vi "AlliGator Fit Decay.vi"(0 "Selected Plot Info + Flag":T13={"Multiplot XY Graph"=refnum, "Mouse Coordinates"={"Horizontal"=0, "Vertical"=0}, "Plot Index"=-1, "Flag"=FALSE}, 1 "Decay Fit Options & Parameters":T2={"SYNC Period"=0.0, "Fit Options"={"Show Fit Residuals"=FALSE, "Fit Model"=enum."1-Exponential", "Residual Type"=enum."Standard", "Max Decay Percentile"=0.0, "Min Decay Percentile"=0.0, "Show Full Decay"=FALSE, "Weights"=enum."Unweighted", "Fitting Method"=enum."Least Square", "Compute Parameter Uncertainties"=FALSE, "Periodic Boundaries"=FALSE, "Model Calculation"=enum."Simulation", "Period"=0.0, "Termination Criteria"={"Max Iterations"=0, "Max Function Calls"=0, "Max Time"=0.0, "Function Tolerance"=0.0, "Parameter Tolerance"=0.0, "Gradient Tolerance"=0.0, "Min Lambda"=0.0, "Max Lambda"=0.0, "Initial Tick Count"=0}, "Offset Resolution"=0.0, "Use Local IRF"=FALSE, "Fitting Algorithm"=enum."Levenberg-Marquardt", "Show Confidence Interval "=TRUE, "Confidence Level"=95.0}, "Fit Parameter Constraints"=[], "MLE Baseline Offset"=0.0, "MLE Baseline Offset Type"=enum."Absolute"} {"Fit Options"."Confidence Level" min=0.0 max=100.0; "Fit Options"."Offset Resolution" min=0.0; "Fit Options"."Period" min=0.0; "Fit Options"."Min Decay Percentile" min=0.0 max=1.0; "Fit Options"."Max Decay Percentile" min=0.0 max=100.0; "Fit Parameter Constraints"."Max Value" format="%#.3g"; "Fit Parameter Constraints"."Min Value" format="%#.3g"}, 5 "Current Decay Name":string, 7 "Current Decay":T16, 9 "Reference Decay":T16, 11 "error in (no error)":errorcluster, 12 "Use Legacy Fitting Approach":bool) -> (2 "Decay Fit Options & Parameters (out)":T2={"SYNC Period"=0.0, "Fit Options"={"Show Fit Residuals"=FALSE, "Fit Model"=enum."1-Exponential", "Residual Type"=enum."Standard", "Max Decay Percentile"=0.0, "Min Decay Percentile"=0.0, "Show Full Decay"=FALSE, "Weights"=enum."Unweighted", "Fitting Method"=enum."Least Square", "Compute Parameter Uncertainties"=FALSE, "Periodic Boundaries"=FALSE, "Model Calculation"=enum."Simulation", "Period"=0.0, "Termination Criteria"={"Max Iterations"=0, "Max Function Calls"=0, "Max Time"=0.0, "Function Tolerance"=0.0, "Parameter Tolerance"=0.0, "Gradient Tolerance"=0.0, "Min Lambda"=0.0, "Max Lambda"=0.0, "Initial Tick Count"=0}, "Offset Resolution"=0.0, "Use Local IRF"=FALSE, "Fitting Algorithm"=enum."Levenberg-Marquardt", "Show Confidence Interval "=TRUE, "Confidence Level"=95.0}, "Fit Parameter Constraints"=[], "MLE Baseline Offset"=0.0, "MLE Baseline Offset Type"=enum."Absolute"} {"Fit Options"."Confidence Level" min=0.0 max=100.0; "Fit Options"."Offset Resolution" min=0.0; "Fit Options"."Period" min=0.0; "Fit Options"."Min Decay Percentile" min=0.0 max=1.0; "Fit Options"."Max Decay Percentile" min=0.0 max=100.0; "Fit Parameter Constraints"."Max Value" format="%#.3g"; "Fit Parameter Constraints"."Min Value" format="%#.3g"}, 3 "Fit Plots":T1, 4 "Best Fit Parameters (All)":dbl[](array[numeric]), 6 "Delta Best Fit Parameters (All)":dbl[](array[numeric]), 8 "R^2":dbl, 10 "Reduced Chi^2":dbl, 13 "Output Plot Names":string[](array[string]), 14 "Fit Output Message":string, 15 "Error Out":errorcluster)   [LabVIEW 2021, in "AlliGator Decay Fit.lvlib"]
doc: "VI implementing single decay fit with either a single or double exponential model with IRF convolution (or in the absence of IRF, without convolution)."
uses:
  AlliGator Decay Fit.lvlib
  <vilib>/Analysis/Matrix/Datatypes/RealMatrix.ctl
  Graphs/XY Graph/XY Graph Selected Plot Info+Flag.ctl
  Graphs/XY Graph/XY Graph Refnum.ctl
  <vilib>/Utility/miscctls.llb/LVPoint32TypeDef.ctl
  Decay Fit Parameter Map/AlliGator Decay Fit Options & Parameters v4.ctl
  Fits/IRF(X)PSED/Decay Fit Options v4.ctl
  Fits/Decay Convolution/Decay Model.ctl
  Fits/Residual Type.ctl
  Fits/IRF(X)PSED/Fit Weights Type v2.ctl
  Fits/Non-linear Fitting Method v2.ctl
  Fits/Fit Calculation Method.ctl
  Fits/Non-linear Fitting Algorithm.ctl
  AlliGator Decay Fit Parameter Constraints 2.ctl
  Fits/IRF(X)PSED/Decay Fit Parameters In List.ctl
  Fits/IRF(X)PSED/MLE Baseline Offset Type.ctl
  Fits/Fit Plots.ctl
  Settings/AlliGator Settings List.ctl
  Fits/Optimal Offset Selection Criterion.ctl
  Globals, Variables, Constants/AlliGator Variables List.ctl
  Fits/IRF(X)PSED/MLE Fit Options.ctl
  Graphs/LabVIEW Plot Interpolation.ctl
  Graphs/Get Plot at Mouse Click (XY Graph)/Get Plot at Mouse Click [AAC].vi
  <vilib>/Utility/error.llb/Error Cluster From Error Code.vi
  Fits/Decay Convolution/LM model function and gradient (1-Exp, Convolved, Periodic, Fixed Parameters) v3.vi
  Fits/Decay Convolution/LM model function and gradient (2-Exp, Convolved, Periodic, Fixed Parameters) v3.vi
  Fits/Abort Fit Global.vi
  <vilib>/ErrorRing/Error Ring.xnode
  Graphs/Graphs.lvlib
  Settings/AlliGator Settings.lvlib
  Graphs/XY Graph/XY Graph Add-Ons.lvlib
  Fits/Fits.lvlib
  Globals, Variables, Constants/AlliGator Globals, Variables & Constants.lvlib
  Time/Time.lvlib
  Strings/Strings.lvlib
  <vilib>/Analysis/Matrix/NI_Matrix.lvlib
  Decay Fit Parameter Map/AlliGator Decay Fit Parameter Map.lvlib
panel:
  in  "Reset Fit Options & Parameters":bool
  out "Covariance":T17
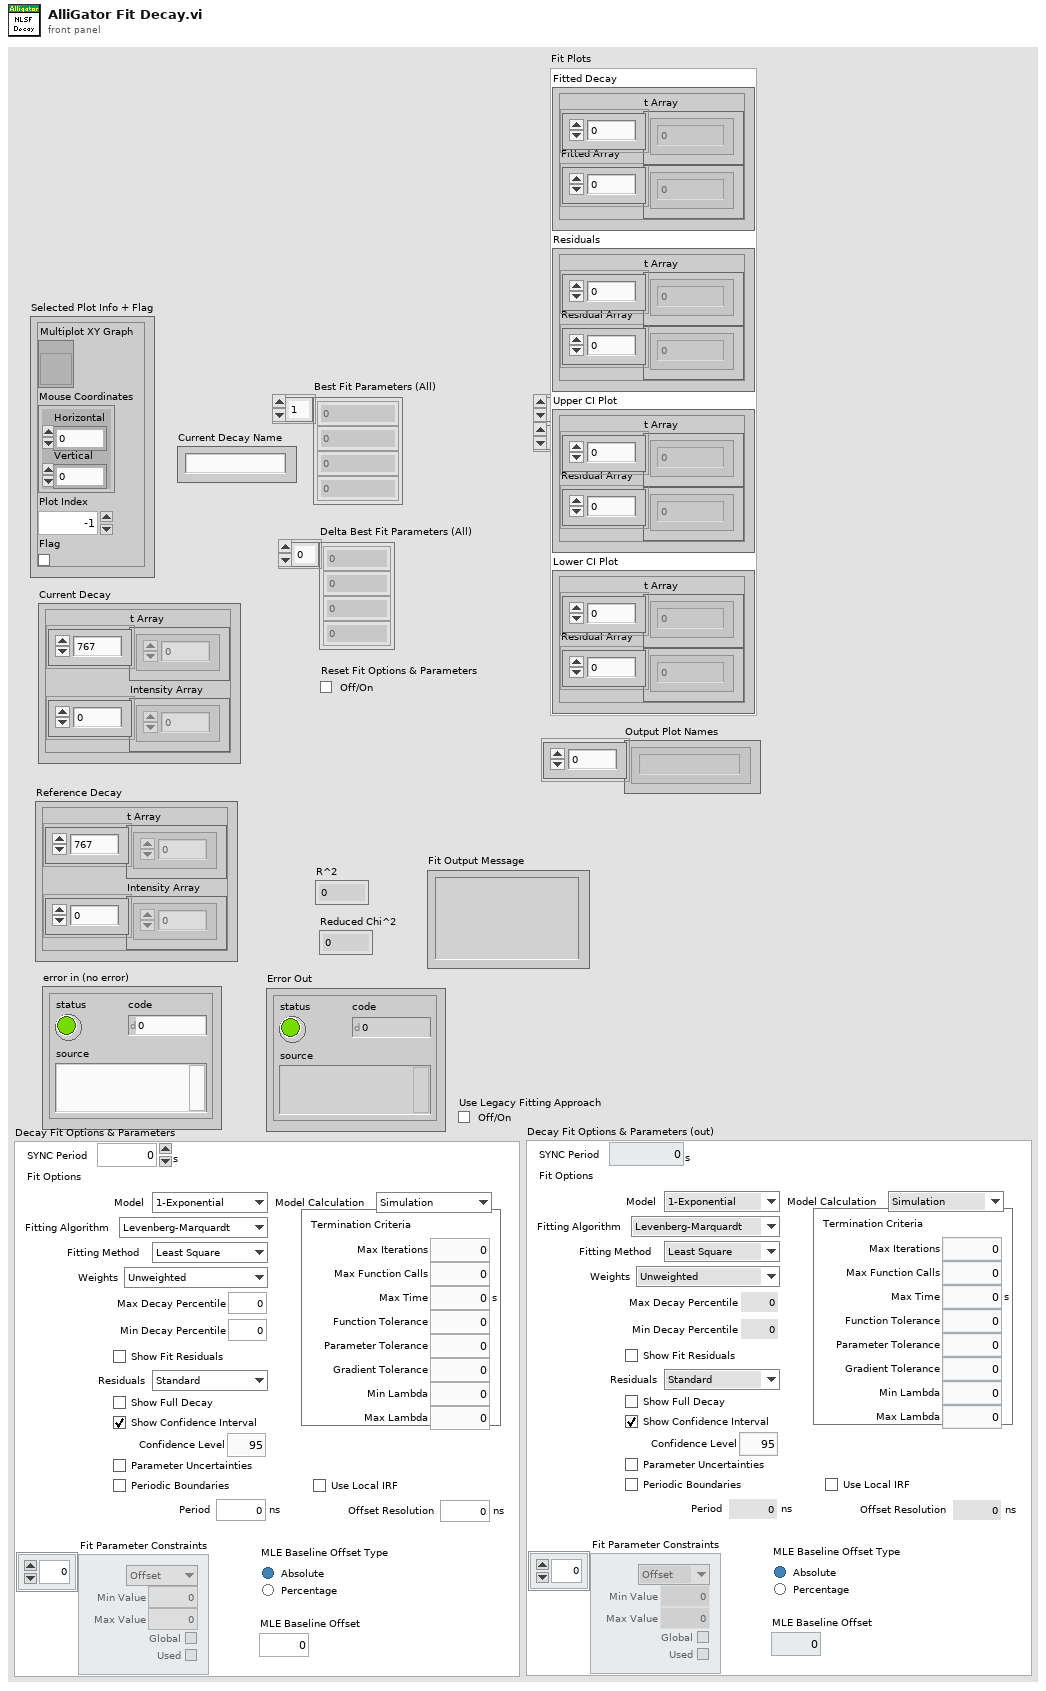
[diagram p1: front panel]
types:
  T1 = typedef "Fits.lvlib/Fit Plots.ctl" = cluster{"Fitted Decay":cluster{"t Array":dbl[], "Fitted Array":dbl[]}, "Residuals":cluster{"t Array":dbl[], "Residual Array":dbl[]}, "Upper CI Plot":cluster{"t Array":dbl[], "Residual Array":dbl[]}, "Lower CI Plot":cluster{"t Array":dbl[], "Residual Array":dbl[]}}
  T2 = typedef "AlliGator Decay Fit Parameter Map.lvlib/AlliGator Decay Fit Options & Parameters v4.ctl" = cluster{"SYNC Period":dbl[unit], "Fit Options":T3, "Fit Parameter Constraints":T10[], "MLE Baseline Offset":dbl, "MLE Baseline Offset Type":T12}
  T3 = typedef "Fits.lvlib/Decay Fit Options v4.ctl" = cluster{"Show Fit Residuals":bool, "Fit Model":T4, "Residual Type":T5, "Max Decay Percentile":dbl, "Min Decay Percentile":dbl, "Show Full Decay":bool, "Weights":T6, "Fitting Method":T7, "Compute Parameter Uncertainties":bool, "Periodic Boundaries":bool, "Model Calculation":T8, "Period":dbl[unit], "Termination Criteria":cluster{"Max Iterations":i32, "Max Function Calls":i32, "Max Time":dbl[unit], "Function Tolerance":dbl, "Parameter Tolerance":dbl, "Gradient Tolerance":dbl, "Min Lambda":dbl, "Max Lambda":dbl, "Initial Tick Count":u32}, "Offset Resolution":dbl[unit], "Use Local IRF":bool, "Fitting Algorithm":T9, "Show Confidence Interval ":bool, "Confidence Level":dbl}
  T4 = typedef "Fits.lvlib/Decay Model.ctl" = enum16{"1-Exponential", "2-Exponentials"}
  T5 = typedef "Fits.lvlib/Residual Type.ctl" = enum16{"Standard", "Normalized", "Reduced"}
  T6 = typedef "Fits.lvlib/Fit Weights Type v2.ctl" = enum16{"Unweighted", "1/Variance (Neyman)", "1/Variance (Pearson)", "Best of All"}
  T7 = typedef "Fits.lvlib/Non-linear Fitting Method v2.ctl" = enum16{"Least Square", "Least Absolute Residual", "Bisquare", "MLE", "-", "Best of All"}
  T8 = typedef "Fits.lvlib/Fit Calculation Method.ctl" = enum16{"Simulation", "Convolution", "Integration"}
  T9 = typedef "Fits.lvlib/Non-linear Fitting Algorithm.ctl" = enum16{"Levenberg-Marquardt", "Trust-Region Dogleg"}
  T10 = typedef "AlliGator Decay Fit.lvlib/AlliGator Decay Fit Parameter Constraints 2.ctl" = cluster{"Fit Parameter":T11, "Min Value":dbl, "Max Value":dbl, "Global":bool, "Used":bool}
  T11 = typedef "Fits.lvlib/Decay Fit Parameters In List.ctl" = enum16{"Offset", "Baseline", "A_1", "tau_1", "A_2", "tau_2"}
  T12 = typedef "Fits.lvlib/MLE Baseline Offset Type.ctl" = enum32{"Absolute", "Percentage"}
  T13 = typedef "XY Graph Add-Ons.lvlib/XY Graph Selected Plot Info+Flag.ctl" = cluster{"Multiplot XY Graph":T14, "Mouse Coordinates":T15, "Plot Index":i32, "Flag":bool}
  T14 = typedef "XY Graph Add-Ons.lvlib/XY Graph Refnum.ctl" = refnum<vi>
  T15 = typedef "LVPoint32TypeDef.ctl" = cluster{"Horizontal":i32, "Vertical":i32}
  T16 = cluster{"t Array":dbl[], "Intensity Array":dbl[]}
  T17 = typedef "NI_Matrix.lvlib/RealMatrix.ctl" = dbl[][]
  T18 = typedef "Fits.lvlib/Optimal Offset Selection Criterion.ctl" = enum16{"Min Chi^2", "Max R^2"}
  T19 = typedef "AlliGator Settings.lvlib/AlliGator Settings List.ctl" = enum16{"GUI:Visible Settings Tab", "GUI:Last Run Version", "Source Image:Use Image Histogram for Contrast", "Source Image:Low Count Pixels Rejection Options", "Source Image:High Count Pixels Rejection Options", "Source Image:Use Image Brightness", "Source Image:Blend Overlay with Image Background", "Source Image:Use Fixed ROI Diameter", "Source Image:ROI Diameter", "Source Image:ROI Center Color", "Source Image:Peak Threshold", "Source Image:Intensity Threshold", "Source Image:Image Binning Options", "Source Image:Image Smoothing Options", "Source Image:Image Histogram Active", "Source Image:Invert Binary Mask", "Source Image:Hot Pixel Removal", "Source Image:Overlay Analyzed ROI Center", "Source Image:Auto-Adjust Contrast", "Source Image:Histogram Lower Percentile", "Source Image:Histogram Upper Percentile", "Source Image:Save Source Image", "Source Image:Scale Bar Options", "Source Image:Image Resolution (Pixel Size)", "Source Image:Flatfield Correction", "Source Image:Show Dead Left Columns Correction", "Source Image:Dead Left Columns Correction", "Source Image:Image Pre-Processing Operations Order", "Source Image:Overlay ROI Median", "Source Image:Median Overlay Color", "Data Information:Gate Width", "Data Information:Nanotime Gate Separation", "Data Information:Macrotime Gate Separation", "Data Information:Gate Step", "Data Information:# Gates", "Data Information:Gate Image Exposure", "Data Information:Gate Image Integration", "Data Information:Gates to Skip", "Data Information:Gates to Keep", "Data Information:Define Gates to", "Data Information:Channel Name", "Data Information:Available Channel Names", "Data Information:Channel Arithmetic", "Data Information:Background File Subtraction", "Data Information:Background File", "Data Information:Background Scaling Factor", "Data Information:Background Pile-up Correction", "Data Information:Background Pixel Well Capacity", "Data Information:Laser Period", "Data Information:SYNC Period", "Data Information:Pile-up Correction", "Data Information:Pixel Well Capacity", "Data Information:Dataset Scaling Factor", "Fluorescence Decay_Decay Pre-Processing:Reverse Gates", "Fluorescence Decay_Decay Pre-Processing:Verbose Decay Pre-Processing", "Fluorescence Decay_Decay Pre-Processing:Use Decay Pre-Processing", "Fluorescence Decay_Decay Pre-Processing:Background Subtraction", "Fluorescence Decay_Decay Pre-Processing:Background Definition Range", "Fluorescence Decay_Decay Pre-Processing:Baseline Subtraction Method", "Fluorescence Decay_Decay Pre-Processing:Decay Pre-Processing Operations Order", "Fluorescence Decay_Decay Pre-Processing:Smoothing Parameter", "Fluorescence Decay_Decay Pre-Processing:Shift Decay", "Fluorescence Decay_Decay Pre-Processing:Decay Shift Parameters", "Fluorescence Decay_Decay Pre-Processing:Fold Decay", "Fluorescence Decay_Decay Pre-Processing:# Folds", "Fluorescence Decay_Decay Pre-Processing:1-Normalize Decay", "Fluorescence Decay_Decay Pre-Processing:[0-1]-Normalize Decay", "Fluorescence Decay_Decay Pre-Processing:Smoothen Decay", "Fluorescence Decay_Decay Pre-Processing:Extrapolate Decay", "Fluorescence Decay_Decay Pre-Processing:Use Periodicity", "Fluorescence Decay_Decay Pre-Processing:Use Cursors", "Fluorescence Decay_Decay Pre-Processing:Tail Fraction", "Fluorescence Decay_Decay Pre-Processing:Head Fraction", "Fluorescence Decay_Decay Pre-Processing:Additional Points", "Fluorescence Decay_Decay Pre-Processing:Straighten Decay", "Fluorescence Decay_Decay Pre-Processing:Constant Background", "Fluorescence Decay_Decay Pre-Processing:Pixel-Normalize Decay", "Fluorescence Decay_Advanced Analysis:Extract IRF instead of Decay", "Fluorescence Decay_Advanced Analysis:IRF Extraction Options", "Fluorescence Decay_Advanced Analysis:IRF Optimization Options", "Fluorescence Decay_Advanced Analysis:Square Pulse Options", "Fluorescence Decay_Advanced Analysis:IRF Order", "Fluorescence Decay_Advanced Analysis:IRF Time Constants", "Fluorescence Decay_Advanced Analysis:Wavelet Analysis Options", "Fluorescence Decay_Advanced Analysis:Average Lifetime Options", "Fluorescence Decay_Fit Options:Fit Options", "Fluorescence Decay_Fit Options:Use Legacy Fitting Approach", "Fluorescence Decay_Fit Options:Use Data Information Laser Period", "Fluorescence Decay_Fit Parameters:Displayed Fit Parameters", "Fluorescence Decay_Fit Parameters:Fit Parameter Constraints", "Fluorescence Decay_Fit Parameters:Export Tabulated Results", "Fluorescence Decay_Fit Parameters:MLE Baseline Offset Type", "Fluorescence Decay_Fit Parameters:MLE Baseline Offset", "Fluorescence Decay_Fit Parameters:Guess Parameter Names", "Fluorescence Decay_Fit Parameters:Guess Parameter Values", "Fluorescence Decay_Fit Parameters:Guess Parameters Options", "Fluorescence Decay_Fit Parameters:Optimal Offset Selection Criterion", "Fluorescence Decay_Styles:Show Last Decay Only", "Fluorescence Decay_Styles:Decay Graph Color Array", "Fluorescence Decay:Decay Graph Active", "Fluorescence Decay Statistics:Min Peak Value", "Fluorescence Decay Statistics:Reject Low Decay Peak Pixels", "Fluorescence Decay Statistics:Reject High Decay Peak Pixels", "Fluorescence Decay Statistics:Max Peak Value", "Time Traces:Use File Timestamp", "Time Traces:Time Step", "Time Traces:Use Intensity Correction File", "Time Traces:Intensity Correction File", "Phasor Plot:Phasor Plot Smoothing Options", "Phasor Plot:Phasor Plot Size", "Phasor Plot:Phasor Plot Graphics Options", "Phasor Plot:Cumulative Phasor Plot", "Phasor Plot:Use Phasor Brightness", "Phasor Plot:Blend Overlay with Phasor Background", "Phasor Plot:Save Phasor Plot", "Phasor Plot:Show References", "Phasor Plot:Phasor Ratio Decay Range", "Phasor Plot:Exponential Fading", "Phasor Plot:Phasor Ratio Reference Colors", "Phasor Plot:Reference Radius", "Phasor Plot:Show Color Map Vertices", "Phasor Plot:Phasor Plot Active", "Phasor Plot:Phasor Ratio Color Map Type", "Phasor Plot:Phasor Ratio Color Map", "Phasor Plot:Phasor Ratio Display Range", "Phasor Plot:Selected Image ROI(s)", "Phasor Plot:All Image ROIs", "Phasor Plot:Selected Phasor Plot ROI(s)", "Phasor Plot:All Phasor Plot ROIs", "Phasor Plot:Phasor Ratio Color-Coded Quantity", "Phasor Plot:Store Phasor Harmonics", "Phasor Plot:Draw Reference Segment", "Phasor Plot:User-Defined Quantity", "Phasor Plot:Color Scale High Color", "Phasor Plot:Color Scale Low Color", "Phasor Plot:Intensity-weighted Phasor Plot", "Phasor Graph:Phasor Frequency", "Phasor Graph:Phasor Ratio Type", "Phasor Graph:Pixel-level Phasor Computation", "Phasor Graph:Save Phasor Graph", "Phasor Graph:Phasor Graph Active", "Phasor Graph:Phasor SDV Options", "Phasor Graph:Intensity-weighted Phasor Graph", "Phasor Graph:Define Shortest Lifetime as", "Phasor Calibration:Use Backup Calibration if needed", "Phasor Calibration:Backup Calibration Type", "Phasor Calibration:Calibration Type", "Phasor Calibration:Calibration Lifetime", "Phasor Calibration:Calibration Map Algorithm", "Single-Exponential Phasor Locus (SEPL):Gate Parameters", "Single-Exponential Phasor Locus (SEPL):User-defined Gate", "Single-Exponential Phasor Locus (SEPL):User-defined IRF", "Single-Exponential Phasor Locus (SEPL):Phasor Parameters", "Single-Exponential Phasor Locus (SEPL):Decay & IRF Parameters", "Single-Exponential Phasor Locus (SEPL):Display Parameters", "Lifetime Analysis:Decay Analysis Parameters", "Lifetime Analysis:Lifetime Map Active", "Plugins:Python Settings", "Miscellaneous:Verbose Mode", "Miscellaneous:Beep after Script", "Miscellaneous:Saved Image File Format", "Miscellaneous:Exported Gate Image Settings", "Miscellaneous:Include Loading in Timing", "Miscellaneous:Verbose Settings Mode", "Miscellaneous:Histogram Options", "Miscellaneous:Beep on Error", "Miscellaneous:# Logical Processors Used", "Miscellaneous:ROI Description Max Characters", "Miscellaneous:Verbose Error Mode", "Miscellaneous:Transparent Mask Color"}
  T20 = typedef "XY Graph Add-Ons.lvlib/XY Graph Plot Data.ctl" = cluster{"X Array":dbl[], "Y Array":dbl[]}
  T21 = typedef "AlliGator Globals, Variables & Constants.lvlib/AlliGator Variables List.ctl" = enum16{"---- GUI ----", "GUI:Initialization Status", "GUI:State Indicators Refnum", "GUI:Original AlliGator Menu Items", "GUI:Current Action Loop State", "GUI:Script in progress", "GUI:Playback", "GUI:Loop Playback", "GUI:Search ROI Used", "GUI:Search ROI", "Decay Graph Max Legend Size", "Intensity Graph Max Legend Size", "Decay Statistics Graph Max Legend Size", "Phasor Graph Max Legend Size", "Phasor Ratio Graph Max Legend Size", "Lifetime Graph Max Legend Size", "---- Files ----", "Files:Export Dataset Frames as Individual Files", "Files:Show Batch Export Help Balloons", "Files:Frames in Dataset", "Files:ptu File Frame Start Indices", "Files:Current Frame in Dataset", "Files:Current Frame Timestamp", "Files:Dataset Loaded", "Files:Dataset Metadata", "Files:Dataset Channel", "Files:Dataset Data Description", "Files:Background Dataset Metadata", "Files:Background Dataset Channel", "Files:Background Dataset Data Description", "Files:Background File Subtraction", "Files:Background File Path", "Files:Background File Pile-up Correction", "Files:Background File Pixel Well Capacity", "Files:Background File Scaling Factor", "Files:Current Dataset Load Settings", "Files:Dataset Path", "Files:ICCD-specific Information", "Files:Macrotime Gate Separation", "------ Python Plugins ------", "Python Plugins:Information", "Python Plugins:Python Session", "Python Plugins:Valid Python Session?", "---- Source Image ----", "Source Image:ROIs", "Source Image:Current ROI", "Source Image:ROI Event Refnum", "X_Source Image:Display Range", "X_Source Image:Palette Information", "X_Source Image:Type of Displayed Image", "X_Time Gate Slider", "Source Image:Palette List", "Source Image:Scale", "Source Image:ROI Overlay Color", "Source Image:Overlay to Erase", "Source Image:Is Displayed Image Accumulated", "Source Image:White Light Image Modified", "Source Image:Mask Image Modified", "---- Image Profile Window ----", "Image Profile:Window Event Refnum", "Image Profile:IntensityType", "Image Profile:Intensity Average Type", "Image Profile:Intensity-weighted SDV", "Image Profile:Box Profile Type", "Image Profile:Window Open", "Image Profile:Plotted Fit Parameter", "------ Phasor Graph -------", "Phasor Graph:Show Line", "---- Phasor Plot ---", "Phasor Plot:Parameters Changed", "Phasor Plot:FLI Dataset Modified since last Calculation", "Phasor Harmonics Data", "Selected Phasor Harmonics", "Phasor Harmonic Manager Event Refnum", "Phasor Plot:ROIs", "Phasor Plot:Current ROI", "Phasor Plot:ROI Event Refnum", "Phasor Plot:Image Reference Points", "Phasor Plot:Computed", "Phasor Plot:Palette Information", "Phasor Plot:Palette List", "Phasor Plot:Phasor Ratio Palette Information", "Phasor Plot:Phasor Ratio Palette List", "Phasor Plot:Image Scale", "Phasor Plot:Image Overlay to Erase", "Phasor Plot:Image Elements to Update", "Phasor Plot:Current Calculation Parameters", "Phasor Plot:Current Calibration Options", "Phasor Plot:Reset Cumulated Phasor Plot", "Phasor Plot:Reference 1", "Phasor Plot:Lifetime Reference 1", "Phasor Plot:Reference 1 Frequency", "Phasor Plot:Reference 2", "Phasor Plot:Lifetime Reference 2", "Phasor Plot:Reference 2 Frequency", "---- Decay Analysis ----", "Number of Selected Decays to Fit", "LS Fit Results", "LAR Fit Results", "BS Fit Results", "Last Decay Max - Min", "Best Fit Parameters", "Best Fit Parameter Names", "Actual Size X", "Actual Size Y", "Binning X", "Binning Y", "Actual # Gates", "Dataset Number", "Gates to...", "Gates Skipped", "Gates to keep", "Gate Step", "Gate Separation", "Reversed Gates", "Pile-up Correction", "Pixel Well Capacity", "Background Subtracted", "Background Subtraction Method", "Background Definition Range", "Background File (deprecated)", "Number of Dataset Accumulated", "Array of Accumulated Dataset Paths", "Do Averaged Datasets", "Destination File Path", "Process Plot Target", "Use 1/D as Phasor Frequency", "---- Decay Fit Parameter Map -----", "Decay Fit Parameter Map:Palette Information", "Decay Fit Parameter Map:Palette List", "Decay Fit Parameter Map:X Resolution", "Decay Fit Parameter Map:Y Resolution", "Decay Fit Parameter Map:Use Decay Fit Result Constraints", "Decay Fit Parameter Map:Decay Fit Result Constraints", "Decay Fit Parameter Map:Decay Fit Result Constraints Applied", "---- Parameter Map ----", "Parameter Map:Palette Information", "Parameter Map:Palette List", "------- Local Decay Window ---------", "Local Decay Graph Window:Event Refnum", "Local Decay Graph Window:Use normalized IRF for convolution", "----- Miscellaneous ----", "Misc:Skippable Dialog Windows Status"}
  T22 = typedef "Fits.lvlib/MLE Fit Options.ctl" = cluster{"MLE Baseline Offset":dbl, "MLE Baseline Offset Type":T12}
  T23 = typedef "Fits.lvlib/Decay Fit Parameter Constraints Arrays.ctl" = cluster{"Parameter Bounds (Fix+Fit)":cluster{"parameter minimum":dbl[], "parameter maximum":dbl[]}, "Fitted Parameters":T11[], "Fixed Parameters":T11[], "Fit Model":T4}
  T24 = typedef "Graphs.lvlib/Plot Range.ctl" = cluster{"X Minimum":dbl, "X Maximum":dbl, "Y Minimum":dbl, "Y Maximum":dbl}
  T25 = cluster{"parameter minimum":dbl[], "parameter maximum":dbl[]}
  T26 = typedef "Fits.lvlib/Non-linear Fit Output v4.ctl" = cluster{"best nonlinear fit":dbl[], "best fit parameters":dbl[], "R^2":dbl, "RMSE":dbl, "error out":errorcluster, "Fitting Method":T27, "number of function calls":i32, "number of iterations":i32, "covariance":T17, "Chi 2":dbl, "DOF":i32, "Fit Convergence Criterion":T28, "Fitting Algorithm":T9, "Weighted Fit":T6, "Gradient":dbl, "|Delta Chi 2|":dbl, "|Delta Chi 2|/Chi 2":dbl, "Max |Delta a| /|a|":dbl, "Lambda":dbl, "RSS":dbl, "AIC":dbl, "BIC":dbl, "Max number of function calls":i32, "Max number of iterations":i32, "IRF":T20, "IRF Normalization Factor":dbl, "Decay Normalization Factor":dbl, "Number of offset fits":i32, "Weighted Chi2":dbl, "Unweighted Chi2":dbl}
  T27 = typedef "Fits.lvlib/Nonlinear Fit Method.ctl" = enum16{"Least Square", "Least Absolute Residual", "Bisquare", "MLE"}
  T28 = typedef "Fits.lvlib/Convergence Criteria.ctl" = enum16{"Continue", "Tolerances Exceeded", "Max Time Exceeded", "Max Iterations Exceeded", "Max Function Evaluations Exceeded", "Scale Range Exceeded"}
  T29 = typedef "AlliGator Decay Fit.lvlib/AlliGator Guess Parameters Options.ctl" = enum16{"Numerically estimated", "User-provided", "User-provided (normalized)", "Last valid fitted parameters"}
  T30 = typedef "Fits.lvlib/Fit Control Data v2.ctl" = cluster{"IRF":T20, "Laser Period":dbl, "SYNC Period":dbl, "Fixed Parameter Names":T11[], "Fixed Parameter Values":dbl[], "Fitted Parameter Names":T11[], "Fit Model":T4}
  T31 = typedef "Graphs.lvlib/LabVIEW Plot Interpolation.ctl" = enum16{"Point (.)", "Stepwise Right (--.)", "Line + Point (\\. /)", "Stepwise Left (.--)", "Stepwise Centered (-.-)", "Stepwise Vertical (|.|)", "Line (-)", "Use Previous Plot's Style"}
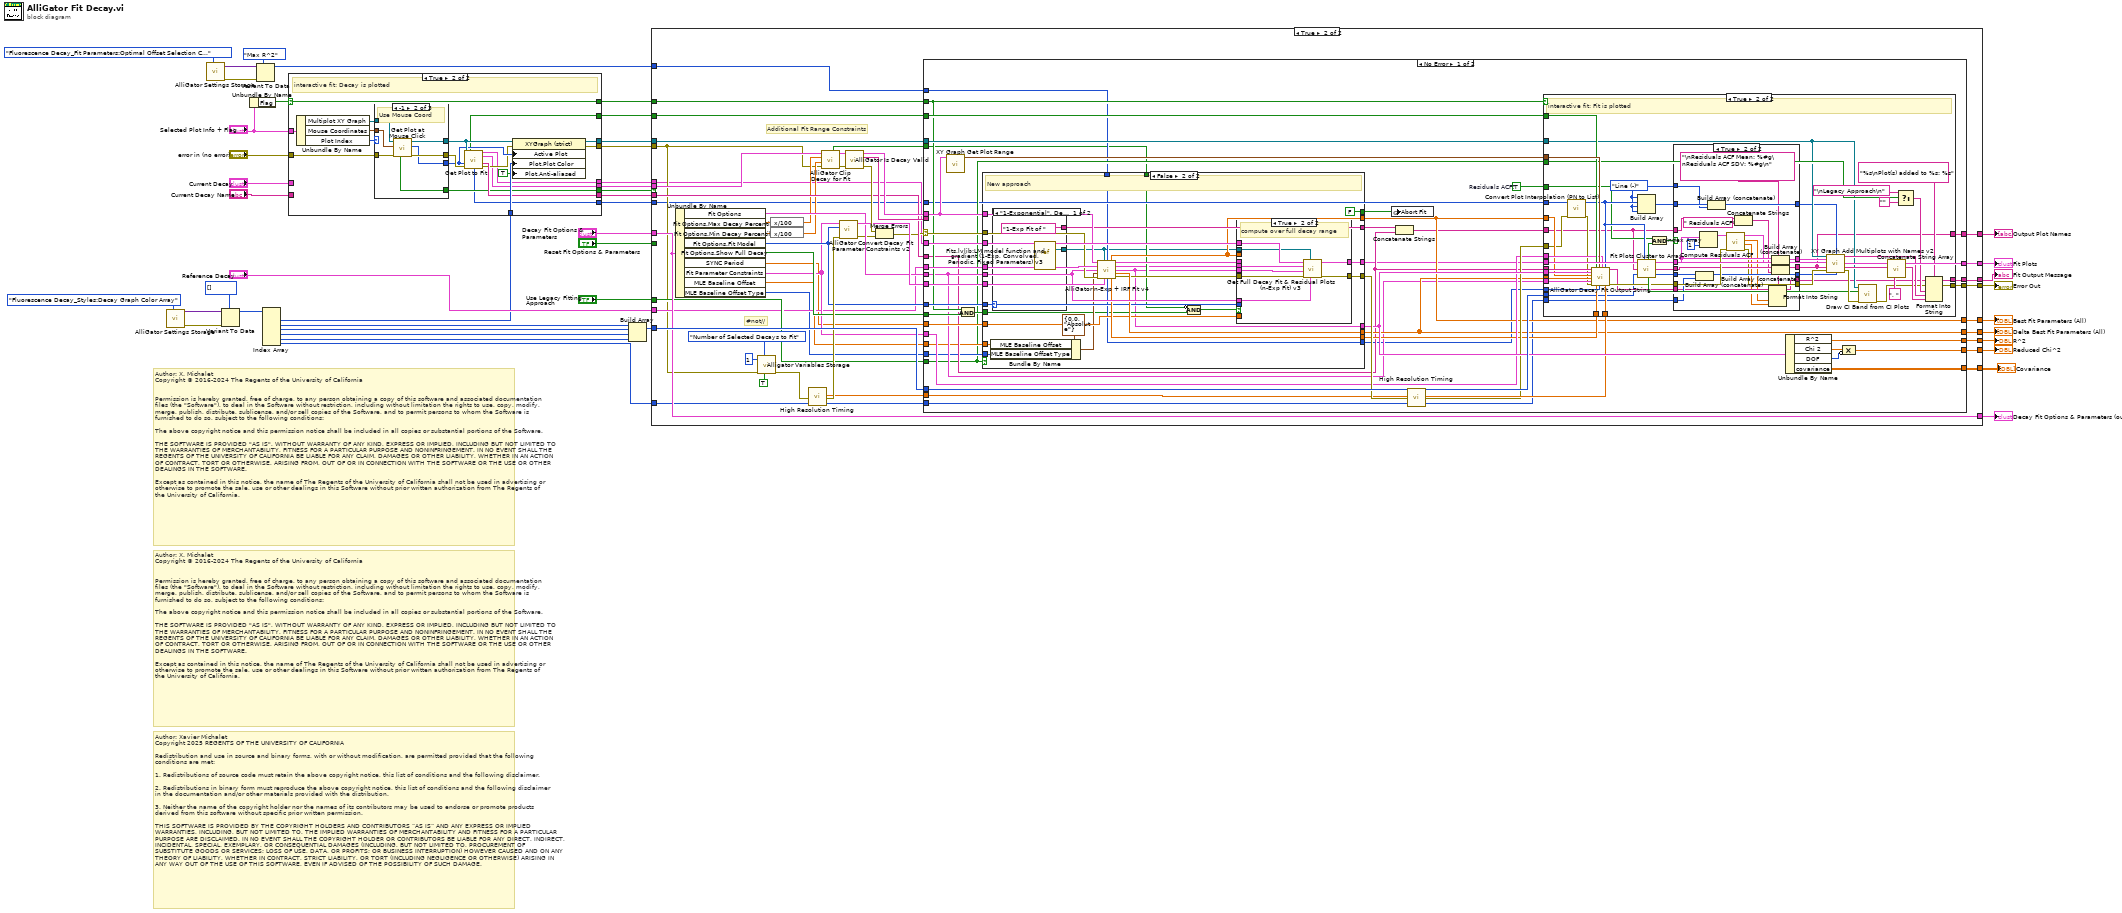
[diagram p0: block diagram]
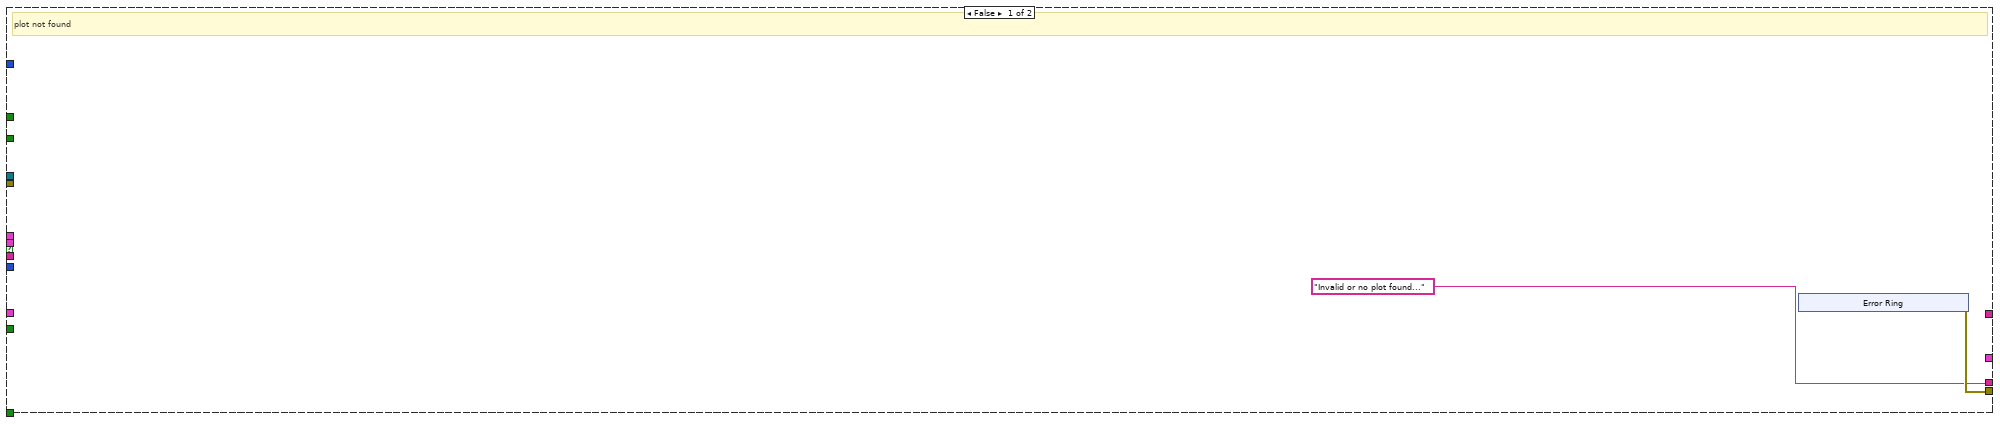
[diagram p2: hidden frame]
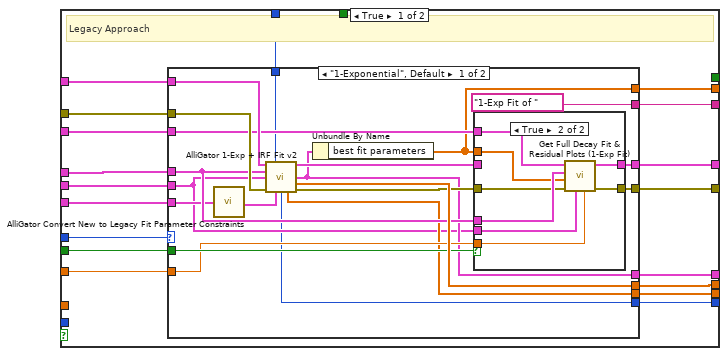
[diagram p5: hidden frame]
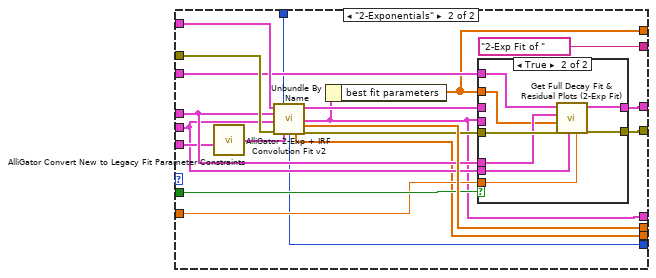
[diagram p7: hidden frame]
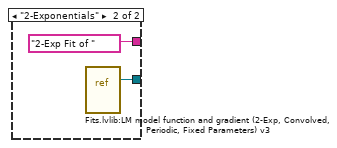
[diagram p9: hidden frame]
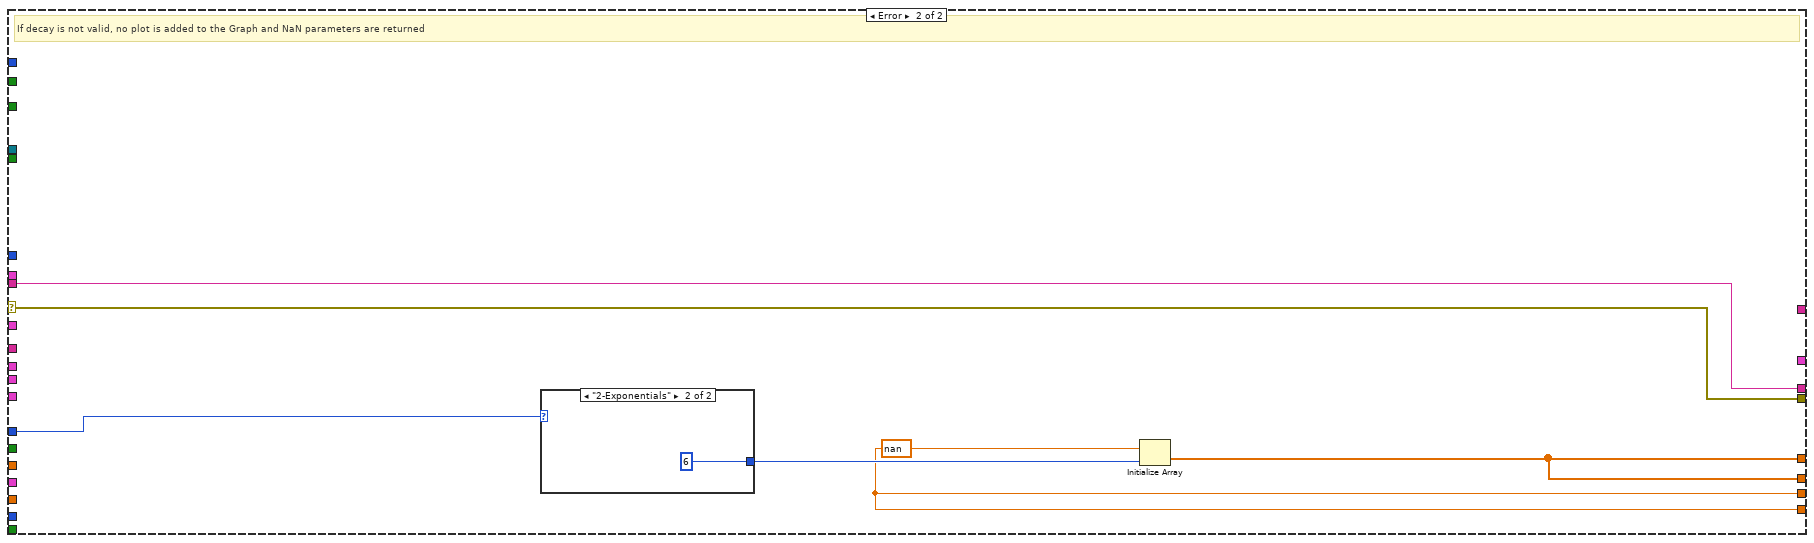
[diagram p11: hidden frame]
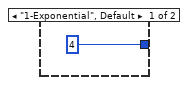
[diagram p12: hidden frame]
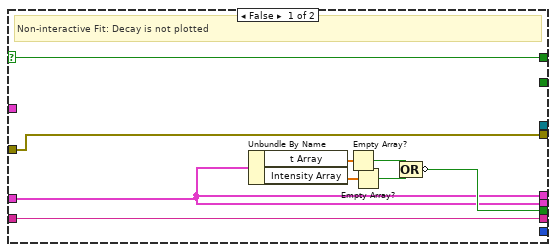
[diagram p13: hidden frame]
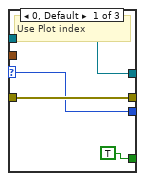
[diagram p14: hidden frame]
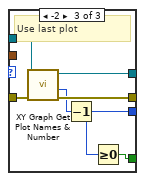
[diagram p15: hidden frame]
diagram:
  # "Author: Xavier Michalet\nCopyright 2025 REGENTS OF THE UNIVERSITY OF CALIFORNIA\n\nRedistribution and use in source and binary forms, with or without modification, are permitted provided that the following conditions are met:\n\n1. Redistributions of source code must retain the above copyright notice, this list of conditions and the following disclaimer.\n\n2. Redistributions in binary form must reproduce the above copyright notice, this list of conditions and the following disclaimer in the documentation and/or other materials provided with the distribution.\n\n3. Neither the name of the copyright holder nor the names of its contributors may be used to endorse or promote products derived from this software without specific prior written permission.\n\nTHIS SOFTWARE IS PROVIDED BY THE COPYRIGHT HOLDERS AND CONTRIBUTORS “AS IS” AND ANY EXPRESS OR IMPLIED WARRANTIES, INCLUDING, BUT NOT LIMITED TO, THE IMPLIED WARRANTIES OF MERCHANTABILITY AND FITNESS FOR A PARTICULAR PURPOSE ARE DISCLAIMED. IN NO EVENT SHALL THE COPYRIGHT HOLDER OR CONTRIBUTORS BE LIABLE FOR ANY DIRECT, INDIRECT, INCIDENTAL, SPECIAL, EXEMPLARY, OR CONSEQUENTIAL DAMAGES (INCLUDING, BUT NOT LIMITED TO, PROCUREMENT OF SUBSTITUTE GOODS OR SERVICES; LOSS OF USE, DATA, OR PROFITS; OR BUSINESS INTERRUPTION) HOWEVER CAUSED AND ON ANY THEORY OF LIABILITY, WHETHER IN CONTRACT, STRICT LIABILITY, OR TORT (INCLUDING NEGLIGENCE OR OTHERWISE) ARISING IN ANY WAY OUT OF THE USE OF THIS SOFTWARE, EVEN IF ADVISED OF THE POSSIBILITY OF SUCH DAMAGE."
  # "Author: X. Michalet\nCopyright © 2016-2024 The Regents of the University of California\n \n\nPermission is hereby granted, free of charge, to any person obtaining a copy of this software and associated documentation files (the \"Software\"), to deal in the Software without restriction, including without limitation the rights to use, copy, modify, merge, publish, distribute, sublicense, and/or sell copies of the Software, and to permit persons to whom the Software is furnished to do so, subject to the following conditions:\n\nThe above copyright notice and this permission notice shall be included in all copies or substantial portions of the Software.\n\nTHE SOFTWARE IS PROVIDED \"AS IS\", WITHOUT WARRANTY OF ANY KIND, EXPRESS OR IMPLIED, INCLUDING BUT NOT LIMITED TO THE WARRANTIES OF MERCHANTABILITY, FITNESS FOR A PARTICULAR PURPOSE AND NONINFRINGEMENT. IN NO EVENT SHALL THE REGENTS OF THE UNIVERSITY OF CALIFORNIA BE LIABLE FOR ANY CLAIM, DAMAGES OR OTHER LIABILITY, WHETHER IN AN ACTION OF CONTRACT, TORT OR OTHERWISE, ARISING FROM, OUT OF OR IN CONNECTION WITH THE SOFTWARE OR THE USE OR OTHER DEALINGS IN THE SOFTWARE.\n\nExcept as contained in this notice, the name of The Regents of the University of California shall not be used in advertising or otherwise to promote the sale, use or other dealings in this Software without prior written authorization from The Regents of the University of California."
  # "Author: X. Michalet\nCopyright © 2016-2024 The Regents of the University of California\n \n\nPermission is hereby granted, free of charge, to any person obtaining a copy of this software and associated documentation files (the \"Software\"), to deal in the Software without restriction, including without limitation the rights to use, copy, modify, merge, publish, distribute, sublicense, and/or sell copies of the Software, and to permit persons to whom the Software is furnished to do so, subject to the following conditions:\n\nThe above copyright notice and this permission notice shall be included in all copies or substantial portions of the Software.\n\nTHE SOFTWARE IS PROVIDED \"AS IS\", WITHOUT WARRANTY OF ANY KIND, EXPRESS OR IMPLIED, INCLUDING BUT NOT LIMITED TO THE WARRANTIES OF MERCHANTABILITY, FITNESS FOR A PARTICULAR PURPOSE AND NONINFRINGEMENT. IN NO EVENT SHALL THE REGENTS OF THE UNIVERSITY OF CALIFORNIA BE LIABLE FOR ANY CLAIM, DAMAGES OR OTHER LIABILITY, WHETHER IN AN ACTION OF CONTRACT, TORT OR OTHERWISE, ARISING FROM, OUT OF OR IN CONNECTION WITH THE SOFTWARE OR THE USE OR OTHER DEALINGS IN THE SOFTWARE.\n\nExcept as contained in this notice, the name of The Regents of the University of California shall not be used in advertising or otherwise to promote the sale, use or other dealings in this Software without prior written authorization from The Regents of the University of California."
  n1 = call "AlliGator Settings Storage.vi"("AlliGator Settings List"=AlliGator_Settings_List."Fluorescence Decay_Styles:Decay Graph Color Array") -> ("Error Out"=w36:errorcluster, "Variant Data out"=w37:variant)  [unwired: 9 in]
  n2 = call "AlliGator Settings Storage.vi"("AlliGator Settings List"=AlliGator_Settings_List."Fluorescence Decay_Fit Parameters:Optimal Offset Selection Criterion") -> ("Error Out"=w10:errorcluster, "Variant Data out"=w9:variant)  [unwired: 9 in]
  n3 = Variant To Data(error in=w36, type=u32[] [] ("appended array"), Variant=w37) -> (data=w34:u32[])  [unwired: 1 out]
  n4 = Unbundle By Name("Selected Plot Info + Flag") -> ("Flag"=w22:bool)
  n5 = Variant To Data(error in=w10, type=Optimal_Offset_Selection_Criterion."Max R^2" ("Optimal Offset Selection Criterion"), Variant=w9) -> (data=w7:T18)  [unwired: 1 out]
  n6 = Index Array(array=w34) -> (element #1=w33:u32, element #2=w3:u32, element #3=w17:u32, element #4=w6:u32, element #5=w2:u32, element #6=w1:u32)  [unwired: 6 in]
  n7 = case shown="True" w22 {
    selector: w22 -> [w47 w58]
    tunnel: w33 -> [_ w71]
    tunnel: "error in (no error)" -> [w54 w70]
    tunnel: [_ w69] -> w31
    tunnel: [w54 w68] -> w30
    tunnel: [w46 w57] -> w29
    tunnel: [w53 w67] -> w28
    tunnel: [_ w66] -> w27
    tunnel: "Current Decay" -> [w46 _]
    tunnel: "Current Decay Name" -> [w53 _]
    tunnel: [w48 w64] -> w24
    tunnel: "Selected Plot Info + Flag" -> [_ w63]
    tunnel: [w47 w58] -> w21
    tunnel: [w46 w56] -> w5
    tunnel: [_ w55] -> w4
    frame False {
      # "Non-interactive Fit: Decay is not plotted"
      n8 = Unbundle By Name(w46) -> ("t Array"=w52:dbl[], "Intensity Array"=w51:dbl[])
      n9 = Empty Array?(array=w52) -> (empty?=w50:bool)
      n10 = Empty Array?(array=w51) -> (empty?=w49:bool)
      n11 = Compound Arithmetic op=OR(w50, w49) -> (invert w48:bool)
    }
    frame True {
      # "interactive fit: Decay is plotted"
      n12 = Unbundle By Name(w63) -> ("Multiplot XY Graph"=w62:T14, "Mouse Coordinates"=w60:T15, "Plot Index"=w61:i32)
      n13 = case shown="-1" w61 {
        selector: w61 -> [w75 _ _]
        tunnel: w70 -> [w78 w85 w91]
        tunnel: [w76 w84 w92] -> w74
        tunnel: [w78 w83 w90] -> w73
        tunnel: [w75 w82 w88] -> w72
        tunnel: [TRUE ("Found?") w81 w87] -> w64
        tunnel: w62 -> [w76 w80 w86]
        tunnel: w60 -> [_ w79 _]
        frame 0, Default {
          # "Use Plot index"
        }
        frame -1 {
          # "Use Mouse Coord"
          n14 = call-poly "Get Plot at Mouse Click.vi"("error in (no error)"=w85, "Mouse Click Coordinates"=w79, "XY Graph in"=w80) -> ("error out"=w83:errorcluster, "Plot at Coordinates"=w82:i32, "XY Graph out"=w84:T14, "Found?"=w81:bool)  [unwired: 2 in, 3 out]
        }
        frame -2 {
          # "Use last plot"
          n15 = call "XY Graph Get Plot Names & Number.vi"("error in (no error)"=w91, "XYGraph in"=w86) -> ("error out"=w90:errorcluster, "# Plots"=w89:i32, "XYGraph out"=w92:T14)  [unwired: 4 in, 3 out]
          n16 = Decrement(x=w89) -> (x-1=w88:i32)
          n17 = Greater Or Equal To 0?(x=w88) -> (x >= 0?=w87:bool)
        }
      }
      n18 = call "Get Plot to Fit.vi"("XYGraph in"=w74, "Plot Index"=w72, "error in (no error)"=w73) -> ("Plot clipped?"=w66:bool, "Full Plot"=w56:T20, "Clipped Plot"=w57:T20, "Plot Name"=w67:string, "Plot Interpolation"=w55:u8, "error out"=w65:errorcluster)  [unwired: 5 in, 2 out]
      n19 = property class="XYGraph (strict)"(reference=w74, error in=w65, "Active Plot"=w72, "Plot.Plot Color"=w71, "Plot.Anti-aliased"=TRUE) -> (reference out=w69:T14, error out=w68:errorcluster)
    }
  }
  n20 = Build Array(w3, w17, w6, w2) -> (w16:u32[])
  n21 = case shown="True" w24 {
    tunnel: [w94 w147] -> w45
    tunnel: ["Invalid or no plot found..." ("Message") w128] -> w44
    tunnel: [_ w146] -> w43
    tunnel: [_ w145] -> w42
    tunnel: [_ w144] -> w41
    tunnel: [_ w143] -> w40
    tunnel: "Reference Decay" -> [_ w112]
    tunnel: w16 -> [_ w142]
    tunnel: [_ w141] -> w32
    tunnel: w31 -> [_ w140]
    tunnel: w30 -> [_ w105]
    tunnel: w29 -> [_ w113]
    tunnel: w28 -> [_ w134]
    tunnel: w27 -> [_ w131]
    tunnel: w21 -> [_ w130]
    tunnel: "Reset Fit Options & Parameters" -> [_ _]
    tunnel: [_ w118] -> w18
    tunnel: "Decay Fit Options & Parameters" -> [_ w118]
    tunnel: "Use Legacy Fitting Approach" -> [_ w117]
    tunnel: [_ w110] -> w12
    tunnel: [_ w109] -> w13
    tunnel: w7 -> [_ w103]
    tunnel: w5 -> [_ w101]
    tunnel: w4 -> [_ w100]
    tunnel: w1 -> [_ w99]
    frame False {
      # "plot not found"
      n22 = xnode "Error Ring"() -> ("error out"=w94:errorcluster)
    }
    frame True {
      # "#not//"
      # "Additional Fit Range Constraints"
      n23 = Unbundle By Name(w118) -> ("Fit Options"=w120:T3, "Fit Options.Max Decay Percentile"=w123:dbl, "Fit Options.Min Decay Percentile"=w115:dbl, "Fit Options.Fit Model"=w122:T4, "Fit Options.Show Full Decay"=w121:bool, "SYNC Period"=w111:dbl[unit], "Fit Parameter Constraints"=w119:T10[], "MLE Baseline Offset"=w108:dbl, "MLE Baseline Offset Type"=w107:T12)
      n24 = call "Alligator Variables Storage.vi"("Get(F)/Set"=TRUE, "AlliGator Variable"=AlliGator_Variables_List."Number of Selected Decays to Fit" ("Alligator Variable"), "Error In"=w105, "Data in"=1) -> ("Error Out"=w124:errorcluster)  [unwired: 5 in, 2 out]
      n25 = expression code="x/100"(w123) -> (w116:dbl)
      n26 = expression code="x/100"(w115) -> (w114:dbl)
      n27 = call "High Resolution Timing.vi"("Error In"=w124) -> ("elapsed (relative) seconds"=w132:dbl, "Error Out"=w133:errorcluster)  [unwired: 16 in, 1 out]
      n28 = call "AlliGator Clip Decay for Fit.vi"("Error In"=w105, "Min Decay Percentile (0)"=w114, "Max Decay Percentile (1)"=w116, "Decay in"=w113) -> ("Error Out"=w138:errorcluster, "Clipped Decay out"=w129:cluster{"t Array":dbl[], "Value Array":dbl[]}, "Full Decay?"=w102:bool)  [unwired: 2 in, 3 out]
      n29 = call "AlliGator Convert Decay Fit Parameter Constraints v2.vi"("Error In"=w133, "Fit Model"=w122, "Fit Parameter Constraints"=w119) -> ("Error Out"=w104:errorcluster, "All Parameter Constraints"=w135:T23)  [unwired: 6 in, 1 out]
      n30 = call "AlliGator Is Decay Valid.vi"("Error In"=w138, "Decay"=w129) -> ("Error Out"=w137:errorcluster, "Message"=w136:string, "Decay (dup)"=w139:cluster{"t Array":dbl[], "Value Array":dbl[]})  [unwired: 6 in, 1 out]
      n31 = Merge Errors(w137, w104) -> (w106:errorcluster)
      n32 = case shown="No Error" w106 {
        selector: w106 -> [w188 w400]
        tunnel: w140 -> [w193 _]
        tunnel: [w192 w400] -> w147
        tunnel: [w166 w397] -> w146
        tunnel: [w165 w397] -> w145
        tunnel: [w183 w396] -> w144
        tunnel: w122 -> [w186 w399]
        tunnel: [w169 w396] -> w143
        tunnel: w112 -> [w191 _]
        tunnel: w121 -> [w190 _]
        tunnel: w101 -> [w189 _]
        tunnel: w139 -> [w179 _]
        tunnel: w134 -> [w162 _]
        tunnel: w120 -> [w164 _]
        tunnel: w136 -> [_ w395]
        tunnel: w142 -> [w187 _]
        tunnel: w135 -> [w185 _]
        tunnel: w119 -> [w170 _]
        tunnel: [w149 _] -> w141
        tunnel: w132 -> [w180 _]
        tunnel: w111 -> [w181 _]
        tunnel: w131 -> [w177 _]
        tunnel: w130 -> [w171 _]
        tunnel: [w174 w395] -> w128
        tunnel: w117 -> [w158 _]
        tunnel: [w153 _] -> w110
        tunnel: [w154 _] -> w109
        tunnel: w108 -> [w160 _]
        tunnel: w107 -> [w159 _]
        tunnel: w103 -> [w157 _]
        tunnel: w102 -> [w152 _]
        tunnel: w100 -> [w151 _]
        tunnel: w99 -> [w148 _]
        frame No Error {
          w150 = TRUE  # Residuals ACF?
          n33 = call "XY Graph Get Plot Range.vi"("Plot in"=w179) -> ("Plot Range"=w178:T24)  [unwired: 10 in]
          n34 = Compound Arithmetic op=AND(w171, w190) -> (w172:bool)
          n35 = case shown="False" w158 {
            tunnel: [w274 w380] -> w154
            tunnel: w191 -> [w291 w379]
            tunnel: w189 -> [w290 w378]
            tunnel: w188 -> [w289 w377]
            tunnel: w186 -> [w288 w367]
            tunnel: w185 -> [w287 w376]
            tunnel: [w286 w375] -> w184
            tunnel: w181 -> [w285 w365]
            tunnel: w179 -> [w284 w374]
            tunnel: [w283 w353] -> w176
            tunnel: w164 -> [w282 w373]
            tunnel: [w281 w372] -> w163
            tunnel: w172 -> [w280 w357]
            tunnel: [w279 w371] -> w167
            tunnel: [w278 w360] -> w166
            tunnel: [w277 w370] -> w165
            tunnel: [_ FALSE ("Abort Fit")] -> w161
            tunnel: w160 -> [_ w364]
            tunnel: w159 -> [_ w363]
            tunnel: w157 -> [w276 w358]
            tunnel: [w275 w359] -> w156
            tunnel: w152 -> [_ w356]
            frame True {
              # "Legacy Approach"
              n36 = case shown="\"1-Exponential\", Default" w288 {
                tunnel: w291 -> [w301 w331]
                tunnel: w289 -> [w311 w341]
                tunnel: ["1-Exp Fit of " ("string") "2-Exp Fit of " ("string")] -> w281
                tunnel: w284 -> [w305 w333]
                tunnel: [w306 w336] -> w274
                tunnel: [w303 w334] -> w286
                tunnel: [w309 w339] -> w277
                tunnel: w280 -> [w308 w338]
                tunnel: w290 -> [w302 w332]
                tunnel: w282 -> [w294 w328]
                tunnel: w287 -> [w300 w330]
                tunnel: [w298 w327] -> w283
                tunnel: w285 -> [w299 w329]
                tunnel: [w297 w325] -> w279
                tunnel: [w296 w326] -> w278
                tunnel: w276 -> [w293 w323]
                tunnel: [w292 w322] -> w275
                frame "1-Exponential", Default {
                  n37 = call "AlliGator Convert New to Legacy Fit Parameter Constraints.vi"("All Parameter Constraints"=w300) -> ("Parameter Bounds"=w295:T25)
                  n38 = call "AlliGator 1-Exp + IRF Fit v2.vi"("Decay"=w305, "Optimal Offset Selection Criterion"=w293, "IRF"=w301, "Fit Options"=w294, "error in (no error)"=w311, "parameter bounds"=w295) -> ("Fit Plots"=w307:T1, "Fit Output"=w298:T26, "Delta Best Fit Parameters"=w309:dbl[], "Guess Parameters Options"=w292:T29, "Guess Parameters"=w297:dbl[], "error out"=w304:errorcluster)  [unwired: 4 in]
                  n39 = Unbundle By Name(w298) -> ("best fit parameters"=w296:dbl[])
                  n40 = case shown="True" w308 {
                    tunnel: w307 -> [w312 _]
                    tunnel: [w312 w317] -> w306
                    tunnel: w301 -> [_ w321]
                    tunnel: w302 -> [_ w320]
                    tunnel: w304 -> [w313 w319]
                    tunnel: [w313 w318] -> w303
                    tunnel: w299 -> [_ w315]
                    tunnel: w294 -> [_ w316]
                    tunnel: w296 -> [_ w314]
                    frame False {
                    }
                    frame True {
                      n41 = call "Get Full Decay Fit & Residual Plots (1-Exp Fit).vi"("Laser Period"=w315, "Fit Options"=w316, "Error In"=w319, "Best Fit Parameters (All)"=w314, "IRF"=w321, "Full Decay"=w320) -> ("Error Out"=w318:errorcluster, "Fit Plots"=w317:T1)  [unwired: 4 in]
                    }
                  }
                }
                frame "2-Exponentials" {
                  n42 = call "AlliGator Convert New to Legacy Fit Parameter Constraints.vi"("All Parameter Constraints"=w330) -> ("Parameter Bounds"=w324:T25)
                  n43 = call "AlliGator 2-Exp + IRF Convolution Fit v2.vi"("Decay"=w333, "Optimal Offset Selection Criterion"=w323, "IRF"=w331, "Fit Options"=w328, "error in (no error)"=w341, "parameter bounds"=w324) -> ("Fit Plots"=w337:T1, "Fit Output"=w327:T26, "Delta Best Fit Parameters"=w339:dbl[], "Guess Parameters Options"=w322:T29, "Guess Parameters"=w325:dbl[], "error out"=w335:errorcluster)  [unwired: 4 in]
                  n44 = Unbundle By Name(w327) -> ("best fit parameters"=w326:dbl[])
                  n45 = case shown="True" w338 {
                    tunnel: w337 -> [w342 _]
                    tunnel: [w342 w347] -> w336
                    tunnel: w335 -> [w343 w351]
                    tunnel: [w343 w350] -> w334
                    tunnel: w332 -> [_ w349]
                    tunnel: w331 -> [_ w348]
                    tunnel: w329 -> [_ w345]
                    tunnel: w328 -> [_ w346]
                    tunnel: w327 -> [_ _]
                    tunnel: w326 -> [_ w344]
                    frame False {
                    }
                    frame True {
                      n46 = call "Get Full Decay Fit & Residual Plots (2-Exp Fit).vi"("Laser Period"=w345, "Fit Options"=w346, "Error In"=w351, "Best Fit Parameters"=w344, "IRF"=w348, "Full Decay"=w349) -> ("Error Out"=w350:errorcluster, "Fit Plots"=w347:T1)  [unwired: 4 in]
                    }
                  }
                }
              }
            }
            frame False {
              # "New approach"
              n47 = Bundle By Name(cluster=T22 {"MLE Baseline Offset"=0.0, "MLE Baseline Offset Type"=enum."Absolute"}, "MLE Baseline Offset"=w364, "MLE Baseline Offset Type"=w363) -> (w361:T22)
              n48 = case shown="\"1-Exponential\", Default" w367 {
                tunnel: ["1-Exp Fit of " ("string") "2-Exp Fit of " ("string")] -> w372
                tunnel: [w381 w383] -> w352
                frame "1-Exponential", Default {
                  n49 = vi-ref "Fits.lvlib:LM model function and gradient (1-Exp, Convolved, Periodic, Fixed Parameters) v3.vi"() -> (w381:refnum<vi>)
                }
                frame "2-Exponentials" {
                  n50 = vi-ref "Fits.lvlib:LM model function and gradient (2-Exp, Convolved, Periodic, Fixed Parameters) v3.vi"() -> (w383:refnum<vi>)
                }
              }
              n51 = call "AlliGator n-Exp + IRF Fit v4.vi"("Decay"=w374, "VI Refnum"=w352, "Optimal Offset Selection Criterion"=w358, "IRF"=w379, "Fit Options"=w373, "MLE Fit Options"=w361, "error in (no error)"=w377, "All Parameter Constraints"=w376) -> ("All unscaled Fit Parameters (w tau)"=w360:dbl[], "Fit Plots"=w369:T1, "Fit Control Data out"=w354:T30, "Fit Output"=w353:T26, "Delta Best Fit Parameters (w tau)"=w370:dbl[], "Guess Parameters Options"=w359:T29, "Guess Parameters"=w371:dbl[], "error out"=w368:errorcluster)
              n52 = Compound Arithmetic op=AND(invert w356, w357) -> (w355:bool)
              n53 = case shown="True" w355 {
                tunnel: w369 -> [w386 _]
                tunnel: [w386 w392] -> w380
                tunnel: w378 -> [_ w391]
                tunnel: w368 -> [w385 w394]
                tunnel: [w385 w393] -> w375
                tunnel: w373 -> [_ w389]
                tunnel: w360 -> [_ _]
                tunnel: w367 -> [_ _]
                tunnel: w365 -> [_ _]
                tunnel: w354 -> [_ w387]
                tunnel: w353 -> [_ w388]
                tunnel: w352 -> [_ w390]
                frame False {
                  # "Use data points used for fit"
                }
                frame True {
                  # "compute over full decay range"
                  n54 = call "Get Full Decay Fit & Residual Plots (n-Exp Fit) v3.vi"("Fit Options"=w389, "VI Refnum"=w390, "Error In"=w394, "Fit Output"=w388, "Fit Control Data"=w387, "Full Decay"=w391) -> ("Error Out"=w393:errorcluster, "Fit Plots"=w392:T1)  [unwired: 4 in]
                }
              }
            }
          }
          n55 = global write "Abort Fit Global.vi" "Abort Fit"(w161) -> ()
          n56 = Concatenate Strings(w163, w162) -> (w155:string)
          n57 = call "High Resolution Timing.vi"("relative seconds (NaN)"=w180, "Error In"=w184) -> ("elapsed (relative) seconds"=w175:dbl, "Error Out"=w173:errorcluster)  [unwired: 15 in, 1 out]
          n58 = case shown="True" w171 {
            tunnel: w193 -> [_ w221]
            tunnel: [w194 w234] -> w192
            tunnel: w187 -> [_ w198]
            tunnel: w178 -> [_ w242]
            tunnel: w177 -> [_ w241]
            tunnel: w162 -> [_ w232]
            tunnel: w176 -> [_ w240]
            tunnel: w165 -> [_ w239]
            tunnel: w164 -> [_ w228]
            tunnel: w170 -> [_ w238]
            tunnel: w175 -> [_ w237]
            tunnel: [_ w233] -> w174
            tunnel: w173 -> [w194 w216]
            tunnel: w156 -> [_ w231]
            tunnel: w167 -> [_ w230]
            tunnel: w166 -> [_ w229]
            tunnel: w154 -> [_ w222]
            tunnel: w158 -> [_ w226]
            tunnel: w155 -> [_ w195]
            tunnel: [_ w204] -> w153
            tunnel: w151 -> [_ w218]
            tunnel: w150 -> [_ w212]
            tunnel: w148 -> [_ w199]
            frame False {
              # "Non-interactive Fit: Fit is not plotted"
            }
            frame True {
              w209 = LabVIEW_Plot_Interpolation."Line (-)" ("element")
              # "interactive fit: Fit is plotted"
              n59 = call "Convert Plot Interpolation (PN to List).vi"("Error In"=w216, "Plot Interpolation (PN)"=w218) -> ("Error Out"=w217:errorcluster, "Plot Interpolation (List)"=w215:T31)  [unwired: 8 in]
              n60 = call "AlliGator Decay Fit Output String.vi"("Plot Name"=w232, "Fit Output"=w240, "All Fit Parameters"=w229, "Delta Best Fit Parameters"=w239, "Fit Options"=w228, "Error In"=w217, "Plot clipped?"=w241, "Guess Parameters"=w230, "(Clipped) Plot Range"=w242, "Guess Parameters Options"=w231, "Fit Parameter Constraints"=w238, "Decay Plot Interpolation"=w215, "CPU (s)"=w237) -> ("Fit Output Message"=w201:string, "Error Out"=w203:errorcluster)  [unwired: 5 in]
              n61 = call "Fit Plots Cluster to Array.vi"("Fit Plots in"=w222, "Plot Interpolation"=w215, "Decay Fit Plot Name"=w195, "Color Array in"=w198) -> ("Residuals Plot?"=w213:bool, "Fit Plot Array"=w207:cluster{"t Array":dbl[], "Fitted Array":dbl[]}[], "Plot Names"=w205:string[], "CI Plots?"=w214:bool, "Color Array out"=w197:u32[])  [unwired: 1 in]
              n62 = Build Array(w209, w215, w209, w209) -> (w210:T31[])
              n63 = And(x=w212, y=w213) -> (x .and. y?=w211:bool)
              n64 = case shown="True" w211 {
                tunnel: w210 -> [w250 w273]
                tunnel: w209 -> [_ w272]
                tunnel: [w250 w271] -> w208
                tunnel: w207 -> [w249 w264]
                tunnel: [w249 w263] -> w206
                tunnel: w205 -> [w248 w260]
                tunnel: [w248 w261] -> w204
                tunnel: w203 -> [w247 w268]
                tunnel: [w247 w256] -> w202
                tunnel: w201 -> [w246 w255]
                tunnel: [w246 w254] -> w200
                tunnel: w199 -> [_ w266]
                tunnel: w197 -> [w245 w267]
                tunnel: [w245 w265] -> w196
                tunnel: w195 -> [_ w259]
                frame False {
                }
                frame True {
                  n65 = Build Array (concatenate)(w267, w266) -> (w265:u32[])
                  n66 = Index Array(array=w264, index=1) -> (element=w269:cluster{"t Array":dbl[], "Fitted Array":dbl[]})
                  n67 = Build Array (concatenate)(w273, w272) -> (w271:T31[])
                  n68 = call "Compute Residuals ACF.vi"("Error In"=w268, "Residual Plot in"=w269) -> ("Error Out"=w256:errorcluster, "ACF SDV"=w251:dbl, "ACF Mean"=w252:dbl, "Residual ACF out"=w262:cluster{"X Array":dbl[], "Y Array":dbl[]})  [unwired: 5 in, 1 out]
                  n69 = Concatenate Strings(w259, " Residuals ACF" ("string")) -> (w257:string)
                  n70 = Format Into String(format string="\nResiduals ACF Mean: %#g\nResiduals ACF SDV: %#g\n" ("Fit Output Message"), initial string=w255, w252, w251) -> (resulting string=w254:string)  [unwired: 1 in, 1 out]
                  n71 = Build Array (concatenate)(w264, w262) -> (w263:cluster{"X Array":dbl[], "Y Array":dbl[]}[])
                  n72 = Build Array (concatenate)(w260, w257) -> (w261:string[])
                }
              }
              n73 = call "XY Graph Add Multiplots with Names v2.vi"("XYGraph in"=w221, "Plots Interpolation (Previous Plot's Style)"=w208, "Array of Plots"=w206, "Array of Plot Names (\"Plot\")"=w204, "error in (no error)"=w202, "Plot Colors (Default)"=w196) -> ("XY Graph Caption (or Label)"=w224:string, "Added Plot Names"=w244:string[], "error out"=w220:errorcluster)  [unwired: 5 in, 2 out]
              n74 = call "Draw CI Band from CI Plots.vi"("error in (no error)"=w220, "CI Plots?"=w214, "XYGraph in"=w221) -> ("error out"=w219:errorcluster)  [unwired: 7 in, 1 out]
              n75 = call "Concatenate String Array.vi"("Separator (TAB)"=", ", "String Array"=w244) -> ("Formatted String"=w235:string)  [unwired: 9 in]
              n76 = Select(t="\nLegacy Approach\n", s=w226, f="") -> (s? t:f=w223:string)
              n77 = Format Into String(format string="%s\nPlot(s) added to %s: %s", initial string=w200, error in=w219, w223, w224, w235) -> (resulting string=w233:string, error out=w234:errorcluster)
            }
          }
          n78 = Unbundle By Name(w176) -> ("R^2"=w183:dbl, "Chi 2"=w182:dbl, "DOF"=w168:i32, "covariance"=w149:T17)
          n79 = Compound Arithmetic op=MULTIPLY(w182, invert w168) -> (w169:dbl)
        }
        frame Error {
          w396 = nan ("element")
          # "If decay is not valid, no plot is added to the Graph and NaN parameters are returned"
          n80 = case shown="\"2-Exponentials\"" w399 {
            tunnel: [4 ("dimension size") 6 ("dimension size")] -> w398
            frame "1-Exponential", Default {
            }
            frame "2-Exponentials" {
            }
          }
          n81 = Initialize Array(w396, w398) -> (w397:dbl[])
        }
      }
    }
  }
  "Error Out" <- w45
  "Fit Output Message" <- w44
  "Best Fit Parameters (All)" <- w43
  "Delta Best Fit Parameters (All)" <- w42
  "R^2" <- w41
  "Reduced Chi^2" <- w40
  "Covariance" <- w32
  "Decay Fit Options & Parameters (out)" <- w18
  "Fit Plots" <- w13
  "Output Plot Names" <- w12
